vi "writeStatesSamples.vi"(0 "Game in":refnum<class "Game.lvclass">, 1 "Start Recording":bool, 2 "Clear":bool, 3 "Dump":bool, 5 "error in (no error)":errorcluster, 6 "RobotModelFolder":string, 8 "uk":dbl[](array[numeric])) -> (14 "Game out":refnum<class "Game.lvclass">, 19 "error out":errorcluster)   [LabVIEW 2021, in "Game.lvclass"]
uses:
  Game.lvclass
  Game.lvclass/Game.ctl
  Team_class/Team.lvclass/Team.ctl
  Object_class/Object.lvclass/Object.ctl
  Robot_class/Robot.lvclass/Robot.ctl
  Read AllyRef.vi
  Team_class/Read RobotRef.vi
  Object_class/Read x.vi
  Object_class/Read y.vi
  Robot_class/Read orientation.vi
  Ally_class/Ally.lvclass
  D:/RoboIme/controle/SSL_AI/Team_class/Team.lvclass
  Robot_class/Robot.lvclass
  D:/RoboIme/controle/SSL_AI/Object_class/Object.lvclass
  Utilities_class/Utilities.lvclass
  <vilib>/ptbypt/NI_PtbyPt.lvlib
panel:
  out "output array":dbl[][](array[numeric])
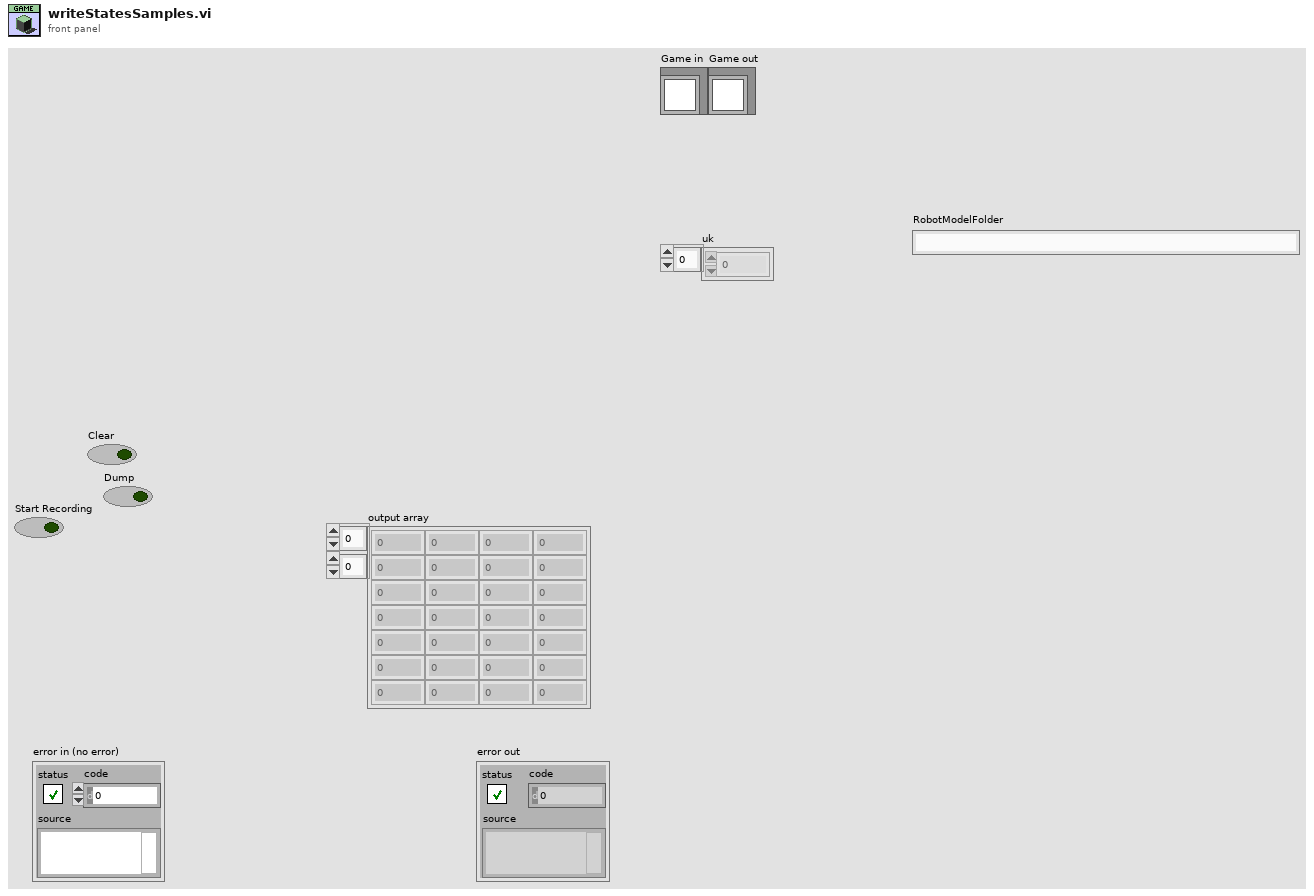
[diagram p1: front panel]
types:
  T1 = cluster{"signal":dbl, "signal":dbl, "signal":dbl}
  T2 = cluster{"signal":dbl, "signal":dbl, "signal":dbl}[]
  T3 = cluster{"x":dbl, "y":dbl, "unwrapped phase":dbl}[]
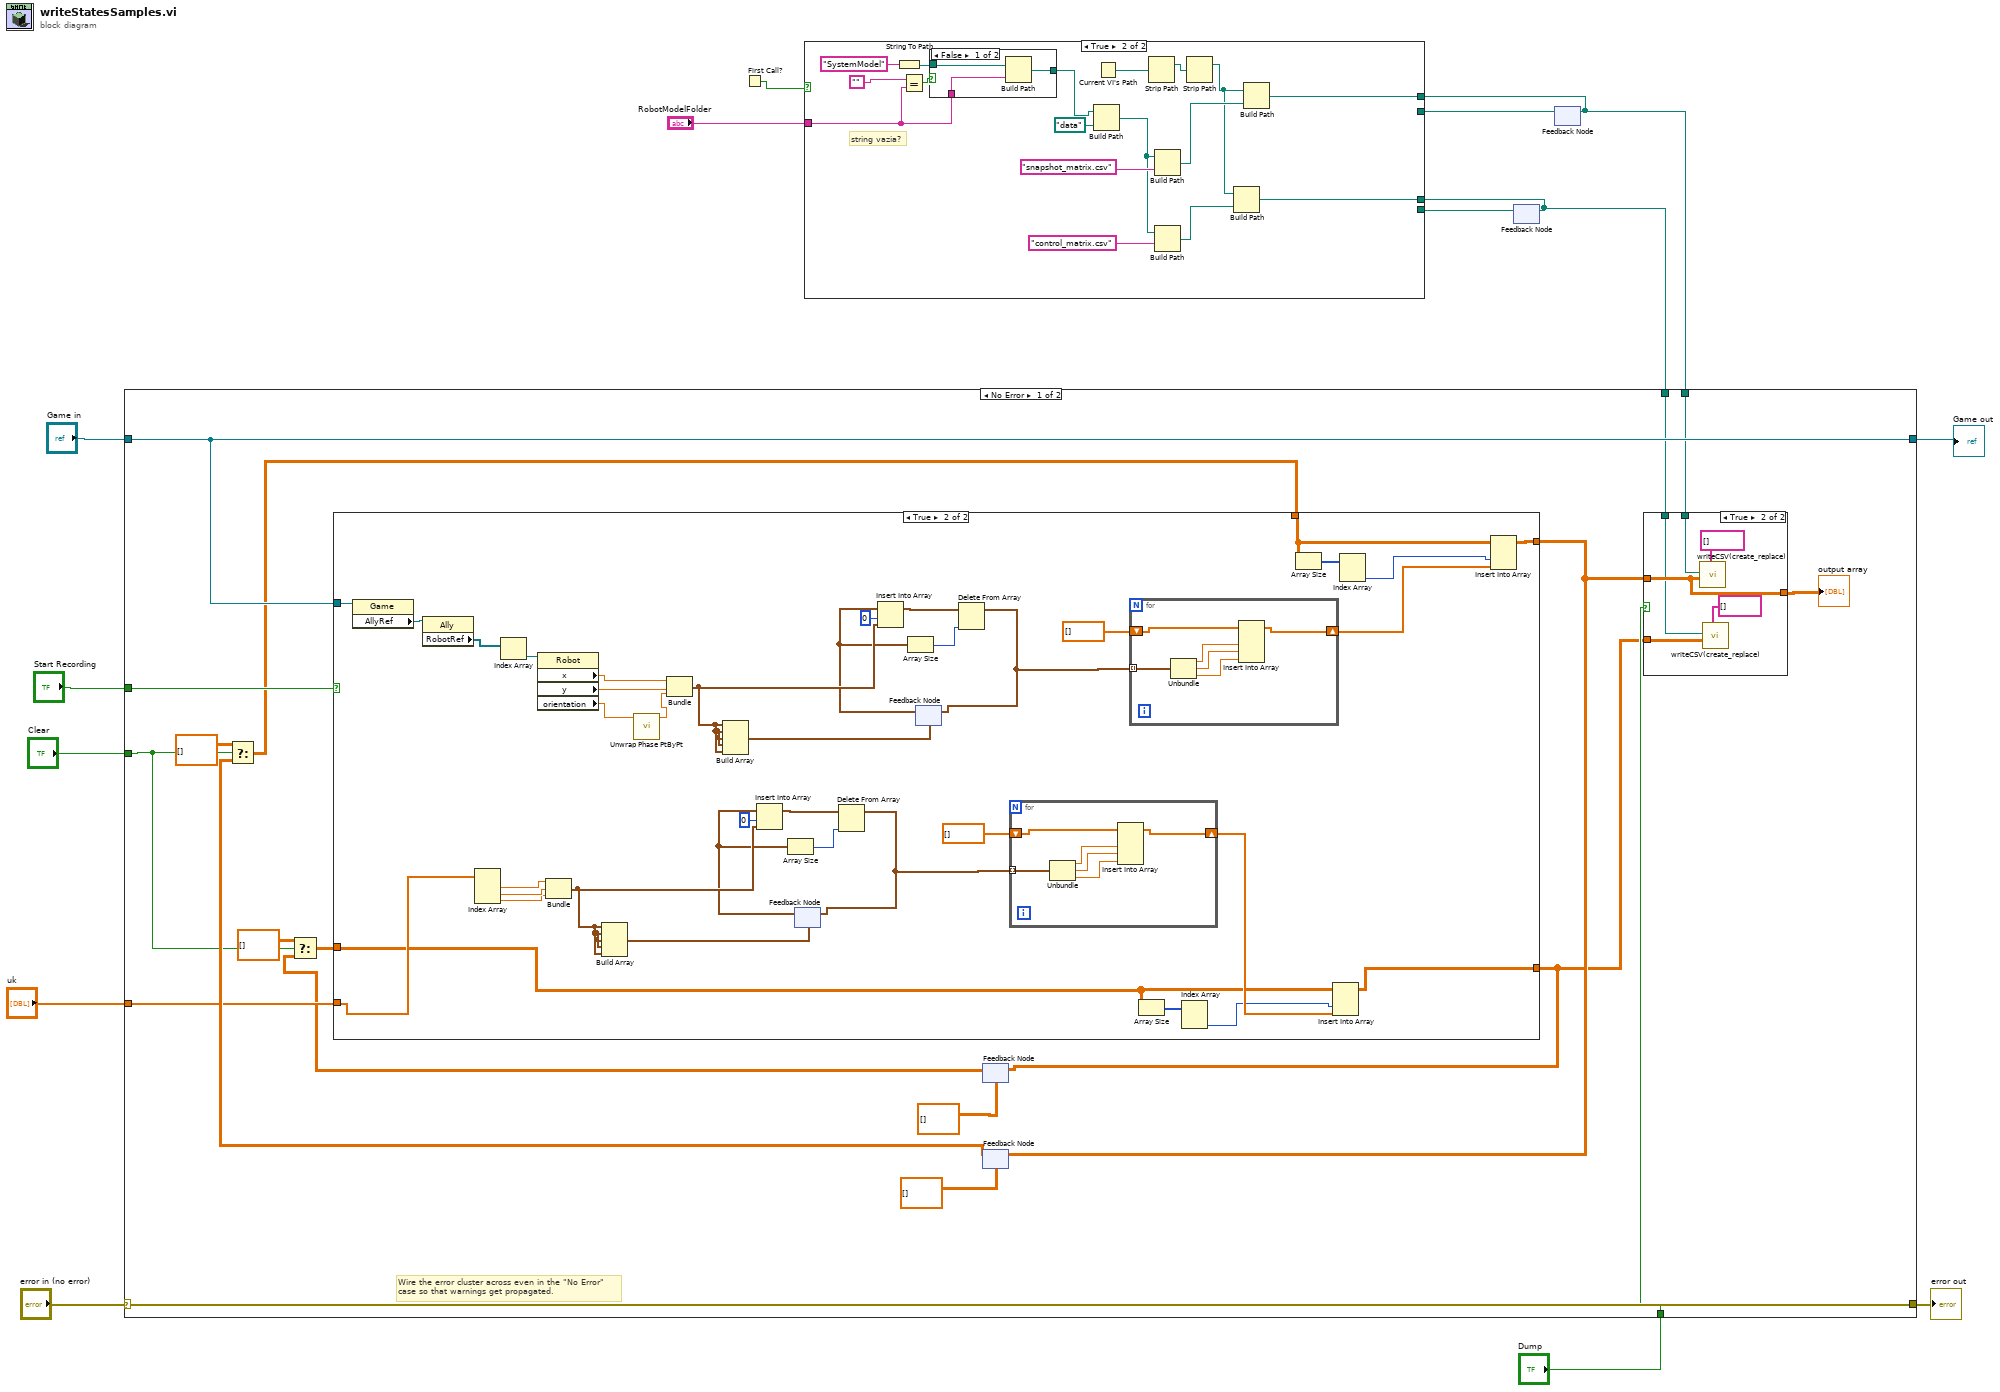
[diagram p0: block diagram]
diagram:
  n1 = First Call?() -> (First Call?: T/F=w10:bool)
  n2 = feedback #1() -> (w4:path)  [unwired: 1 in]
  n3 = feedback #2() -> (w8:path)  [unwired: 1 in]
  n4 = case shown="True" w10 {
    tunnel: [w16 w31] -> w6
    tunnel: "RobotModelFolder" -> [_ w24]
    tunnel: w8 -> [w16 _]
    tunnel: [w15 w20] -> w3
    tunnel: w4 -> [w15 _]
    frame False {
      # "só precisa calcular o path na 1° iteração"
    }
    frame True {
      # "string vazia?"
      n5 = String To Path(string="SystemModel" ("name or relative path")) -> (path=w25:path)
      n6 = Equal?(x="", y=w24) -> (x = y?=w28:bool)
      n7 = case shown="False" w28 {
        tunnel: w24 -> [w36 _]
        tunnel: [w35 w37] -> w19
        tunnel: w25 -> [w34 w37]
        frame False {
          n8 = Build Path(base path=w34, name or relative path=w36) -> (appended path=w35:path)
        }
        frame True {
        }
      }
      n9 = Build Path(base path=w19, name or relative path=path "data") -> (appended path=w17:path)
      n10 = Current VI's Path() -> (path=w33:path)
      n11 = Strip Path(path=w33) -> (stripped path=w32:path)  [unwired: 1 out]
      n12 = Build Path(base path=w17, name or relative path="snapshot_matrix.csv") -> (appended path=w29:path)
      n13 = Build Path(base path=w17, name or relative path="control_matrix.csv") -> (appended path=w22:path)
      n14 = Strip Path(path=w32) -> (stripped path=w21:path)  [unwired: 1 out]
      n15 = Build Path(base path=w21, name or relative path=w22) -> (appended path=w20:path)
      n16 = Build Path(base path=w21, name or relative path=w29) -> (appended path=w31:path)
    }
  }
  n17 = case shown="No Error" "error in (no error)" {
    selector: "error in (no error)" -> [w56 w117]
    tunnel: [w56 w117] -> w13
    tunnel: [w55 w116] -> w1
    tunnel: "Game in" -> [w55 w116]
    tunnel: "Start Recording" -> [w53 _]
    tunnel: "Clear" -> [w43 _]
    tunnel: "Dump" -> [w50 _]
    tunnel: w6 -> [w49 _]
    tunnel: "uk" -> [w45 _]
    tunnel: w3 -> [w39 _]
    frame No Error {
      # "Wire the error cluster across even in the \"No Error\"\ncase so that warnings get propagated."
      n18 = feedback #3(dbl[][] [] ("appended array")) -> (w42:dbl[][])
      n19 = Select(t=dbl[][] [], s=w43, f=w42) -> (s? t:f=w40:dbl[][])
      n20 = feedback #4(dbl[][] [] ("appended array")) -> (w46:dbl[][])
      n21 = Select(t=dbl[][] [], s=w43, f=w46) -> (s? t:f=w51:dbl[][])
      n22 = case shown="True" w53 {
        tunnel: w55 -> [_ w103]
        tunnel: [w65 w90] -> w48
        tunnel: w51 -> [w65 w89]
        tunnel: w45 -> [_ w75]
        tunnel: w40 -> [w64 w71]
        tunnel: [w64 w70] -> w38
        frame False {
        }
        frame True {
          n23 = property class="Game"(reference=w103) -> ("AllyRef"=w102:refnum<class "Ally.lvclass">)  [unwired: 1 in, 2 out]
          n24 = property class="Ally"(reference=w102) -> ("RobotRef"=w101:refnum<class "Robot.lvclass">[])  [unwired: 1 in, 2 out]
          n25 = Index Array(array=w75) -> (element #1=w74:dbl, element #2=w73:dbl, element #3=w72:dbl)  [unwired: 3 in]
          n26 = Index Array(array=w101) -> (element=w100:refnum<class "Robot.lvclass">)  [unwired: 1 in]
          n27 = property class="Robot"(reference=w100) -> ("x"=w67:dbl, "y"=w66:dbl, "orientation"=w69:dbl)  [unwired: 1 in, 2 out]
          n28 = Bundle("signal"=w74, "signal"=w73, "signal"=w72) -> (w85:T1)  [unwired: 1 in]
          n29 = Build Array(w85, w85, w85, w85, w85) -> (w83:T2)
          n30 = call <vilib>:"Unwrap Phase PtByPt.vi"("phase"=w69) -> ("unwrapped phase"=w68:dbl)  [unwired: 10 in]
          n31 = Bundle("x"=w67, "y"=w66, "unwrapped phase"=w68) -> (w98:cluster{"x":dbl, "y":dbl, "unwrapped phase":dbl})  [unwired: 1 in]
          n32 = Build Array(w98, w98, w98, w98, w98) -> (w96:T3)
          n33 = feedback #5(w83) -> (w82:T2)
          n34 = Insert Into Array(array=w82, index=0, new element=w85) -> (w84:T2)
          n35 = Array Size(array=w82) -> (size(s)=w81:i32)
          n36 = Delete From Array(array=w84, index=w81) -> (array with subset deleted=w80:T2)  [unwired: 1 in, 1 out]
          n37 = feedback-in #5(w80) -> ()
          n38 = feedback #6(w96) -> (w95:T3)
          n39 = Insert Into Array(array=w95, index=0, new element=w98) -> (w97:T3)
          n40 = Array Size(array=w95) -> (size(s)=w94:i32)
          n41 = Delete From Array(array=w97, index=w94) -> (array with subset deleted=w93:T3)  [unwired: 1 in, 1 out]
          n42 = feedback-in #6(w93) -> ()
          n43 = for {
            tunnel: w80 -> [w109] mode=indexing
            shift-right: [w107] -> w78
            shift-left: dbl[] [] ("appended array") -> [w108]
            n44 = Unbundle(w109) -> ("signal"=w106:dbl, "signal"=w105:dbl, "signal"=w104:dbl)
            n45 = Insert Into Array(array=w108, new element #1=w106, new element #2=w105, new element #3=w104) -> (w107:dbl[])  [unwired: 1 in]
          }
          n46 = for {
            tunnel: w93 -> [w115] mode=indexing
            shift-right: [w113] -> w91
            shift-left: dbl[] [] ("appended array") -> [w114]
            n47 = Unbundle(w115) -> ("x"=w112:dbl, "y"=w111:dbl, "unwrapped phase"=w110:dbl)
            n48 = Insert Into Array(array=w114, new element #1=w112, new element #2=w111, new element #3=w110) -> (w113:dbl[])  [unwired: 1 in]
          }
          n49 = Array Size(array=w71) -> (size(s)=w77:i32[])
          n50 = Index Array(array=w77) -> (element #2=w76:i32)  [unwired: 2 in, 1 out]
          n51 = Array Size(array=w89) -> (size(s)=w88:i32[])
          n52 = Insert Into Array(array=w71, index (col)=w76, new element=w78) -> (w70:dbl[][])  [unwired: 1 in]
          n53 = Index Array(array=w88) -> (element #2=w87:i32)  [unwired: 2 in, 1 out]
          n54 = Insert Into Array(array=w89, index (col)=w87, new element=w91) -> (w90:dbl[][])  [unwired: 1 in]
        }
      }
      n55 = feedback-in #3(w38) -> ()
      n56 = feedback-in #4(w48) -> ()
      n57 = case shown="True" w50 {
        tunnel: w49 -> [_ w63]
        tunnel: w48 -> [w57 w62]
        tunnel: [w57 w62] -> w47
        tunnel: w39 -> [_ w59]
        tunnel: w38 -> [_ w58]
        frame False {
        }
        frame True {
          n58 = call "writeCSV(create_replace).vi"("Header"=string[] [], "Array"=w62, "file path (use dialog)"=w63) -> ()  [unwired: 7 in, 2 out]
          n59 = call "writeCSV(create_replace).vi"("Header"=string[] [], "Array"=w58, "file path (use dialog)"=w59) -> ()  [unwired: 7 in, 2 out]
        }
      }
      "output array" <- w47
    }
    frame Error {
    }
  }
  "error out" <- w13
  "Game out" <- w1
  n60 = feedback-in #1(w3) -> ()
  n61 = feedback-in #2(w6) -> ()
